vi "RevBinary.vi"(1 "Binary":u8) -> (0 "Rev Binary":u32)   [LabVIEW 2012]
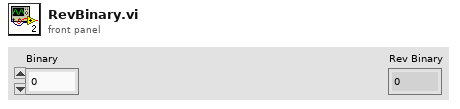
[diagram p1: front panel]
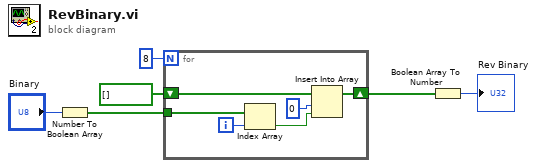
[diagram p0: block diagram]
diagram:
  n1 = Number To Boolean Array(number="Binary") -> (Boolean array=w6:bool[])
  n2 = for {
    N: 8 -> [_]
    tunnel: w6 -> [w11]
    shift-right: [w9] -> w3
    shift-left: bool[] [] -> [w8]
    i -> [w12]
    n3 = Index Array(array=w11, index=w12) -> (element=w10:bool)
    n4 = Insert Into Array(array=w8, index=0, new element=w10) -> (w9:bool[])
  }
  n5 = Boolean Array To Number(Boolean array=w3) -> (number=→"Rev Binary":u32)
